vi "ID_REG.vi"(0 "milliseconds to wait":u32, 1 "Coerce?":bool, 2 "History Data in":dbl[](array[numeric]), 5 "element":T4, 7 "Default værdier":T2, 9 "SP":dbl, 12 "History Data":dbl[](array[numeric]), 13 "Tout":dbl, 14 "ID?":bool) -> (4 "Cluster":T3, 6 "History Data 2":dbl[](array[numeric]), 8 "Tout out":dbl, 15 "P I D":T1)   [LabVIEW 2022 SP3]
uses:
  TypeDefs/P_I_D_Data_type.ctl
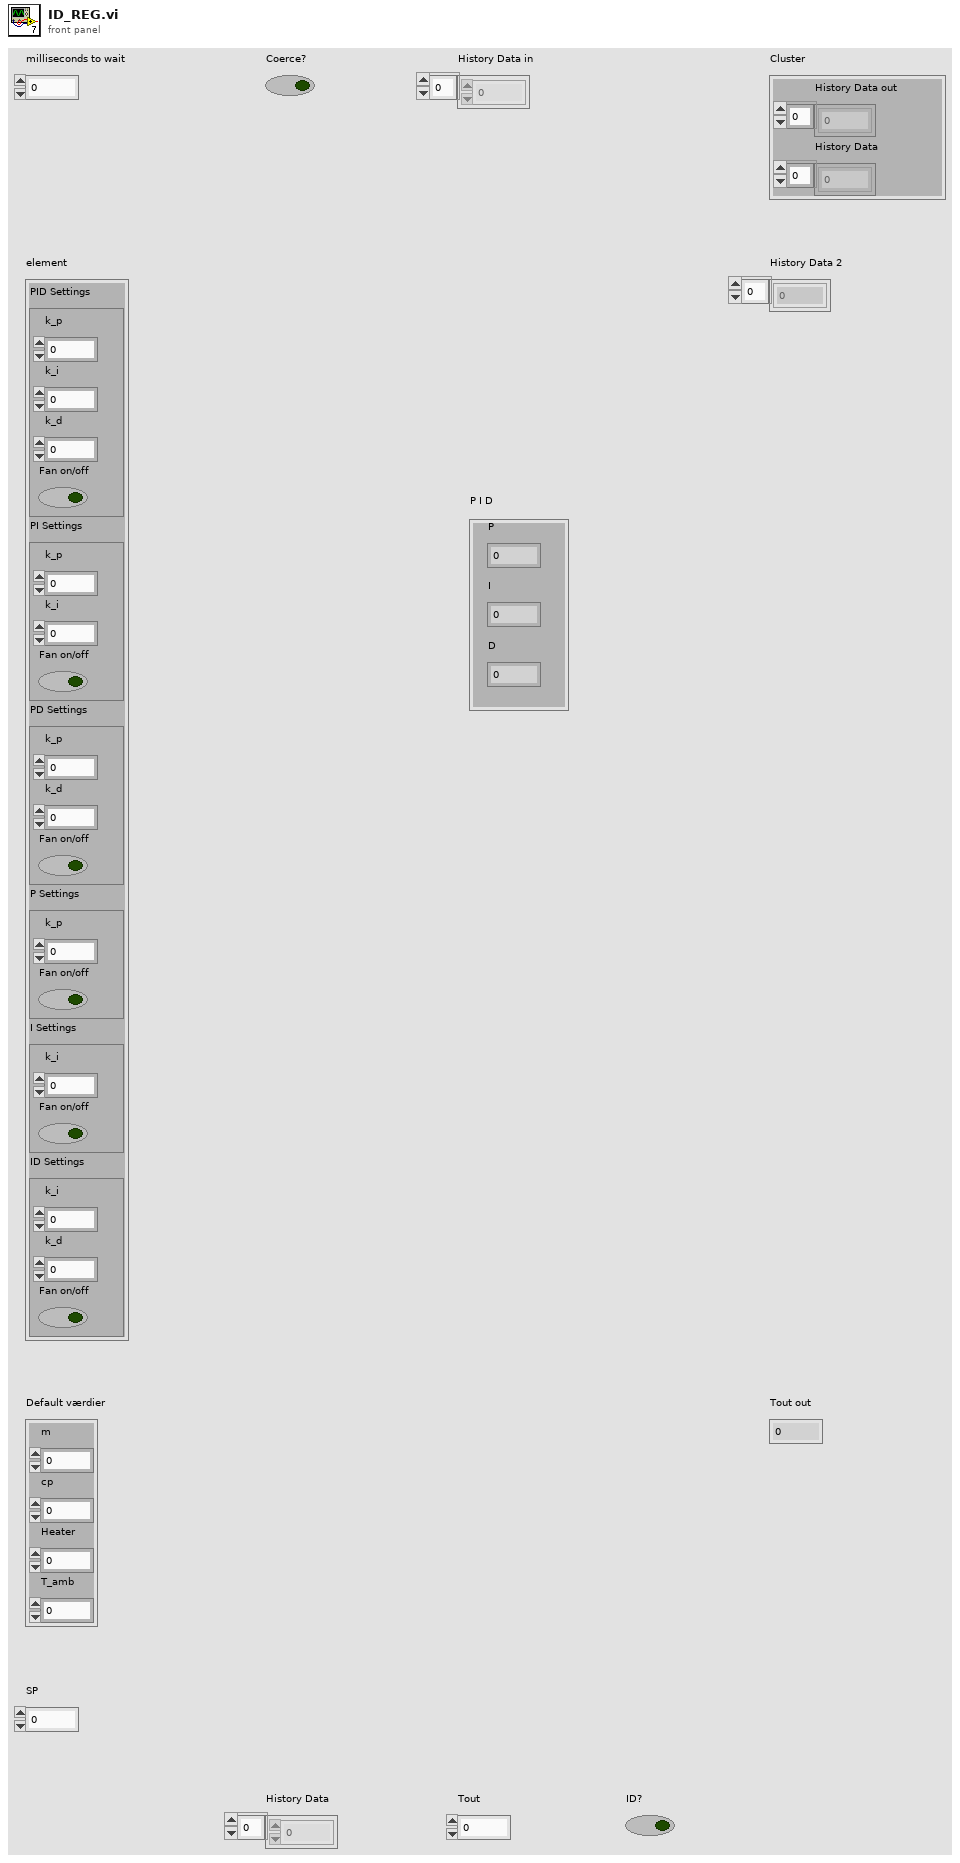
[diagram p1: front panel]
types:
  T1 = typedef "P_I_D_Data_type.ctl" = cluster{"P":dbl, "I":dbl, "D":dbl}
  T2 = cluster{"m":dbl, "cp":dbl, "Heater":dbl, "T_amb":dbl}
  T3 = cluster{"History Data out":dbl[], "History Data":dbl[]}
  T4 = cluster{"PID Settings":cluster{"k_p":dbl, "k_i":dbl, "k_d":dbl, "Fan on/off":bool}, "PI Settings":cluster{"k_p":dbl, "k_i":dbl, "Fan on/off":bool}, "PD Settings":cluster{"k_p":dbl, "k_d":dbl, "Fan on/off":bool}, "P Settings":cluster{"k_p":dbl, "Fan on/off":bool}, "I Settings":cluster{"k_i":dbl, "Fan on/off":bool}, "ID Settings":cluster{"k_i":dbl, "k_d":dbl, "Fan on/off":bool}}
  T5 = enum16{"I_REG", "ID_REG", "P_REG", "PI_REG", "PD_REG", "PID_REG"}
  T6 = cluster{"History Data in":dbl[], "History Data":dbl[]}
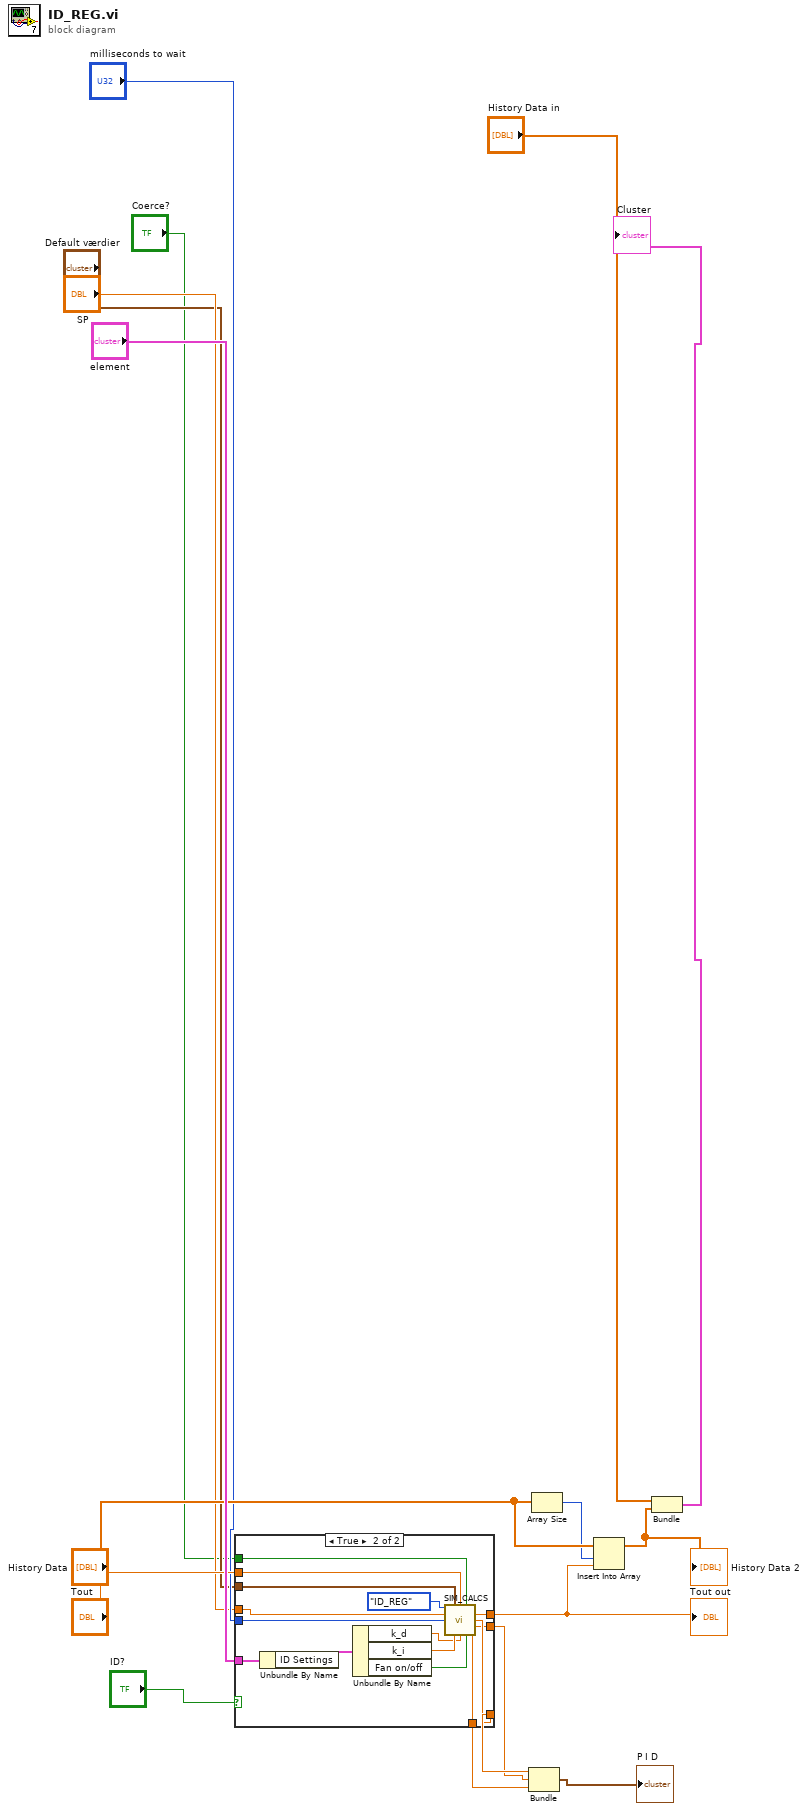
[diagram p0: block diagram]
diagram:
  n1 = case shown="True" "ID?" {
    tunnel: "Tout" -> [_ w31]
    tunnel: "Default værdier" -> [_ w30]
    tunnel: [_ w28] -> w10
    tunnel: "milliseconds to wait" -> [_ w25]
    tunnel: "Coerce?" -> [_ w24]
    tunnel: "SP" -> [_ w23]
    tunnel: "element" -> [_ w22]
    tunnel: [_ w20] -> w4
    tunnel: [_ w19] -> w3
    tunnel: [_ w18] -> w2
    frame False {
    }
    frame True {
      n2 = Unbundle By Name(w22) -> ("ID Settings"=w27:cluster{"k_i":dbl, "k_d":dbl, "Fan on/off":bool})
      n3 = Unbundle By Name(w27) -> ("k_d"=w21:dbl, "k_i"=w32:dbl, "Fan on/off"=w29:bool)
      n4 = call "SIM_CALCS.vi"("Regulation type"=T5."ID_REG", "Default værdier"=w30, "Tout in"=w31, "Coerce?"=w24, "SP"=w23, "milliseconds to wait"=w25, "k_i"=w32, "k_d"=w21, "Fan on/off"=w29) -> ("Tout out"=w28:dbl, "P"=w20:dbl, "I"=w19:dbl, "D"=w18:dbl)  [unwired: 2 in, 1 out]
    }
  }
  "Tout out" <- w10
  n5 = Bundle("P"=w4, "I"=w3, "D"=w2) -> (→"P I D":cluster{"P":dbl, "I":dbl, "D":dbl})  [unwired: 1 in]
  n6 = Array Size(array="History Data") -> (size(s)=w12:i32)
  n7 = Insert Into Array(array="History Data", index=w12, new element=w10) -> (w11:dbl[])
  "History Data 2" <- w11
  n8 = Bundle("History Data in"="History Data in", "History Data"=w11) -> (→"Cluster":T6)  [unwired: 1 in]
